vi "Build Slide Info.vi"(8 "error in (no error)":errorcluster, 11 "Parse Presentation in":refnum<class "Parse Presentation.lvclass">) -> (0 "error out":errorcluster, 3 "Parse Presentation out":refnum<class "Parse Presentation.lvclass">)   [LabVIEW 2015, in "Parse Presentation.lvclass"]
uses:
  Parse Presentation.lvclass
  Slide Info..cluster.ctl
  Parse Presentation.lvclass/Parse Presentation.ctl
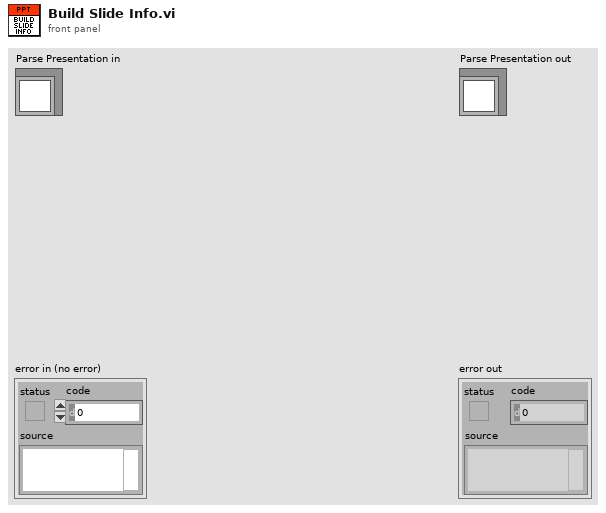
[diagram p1: front panel]
types:
  T1 = typedef "Parse Presentation.lvclass/Slide Info..cluster.ctl" = cluster{"Slide":i32, "Text":string, "Images":string}
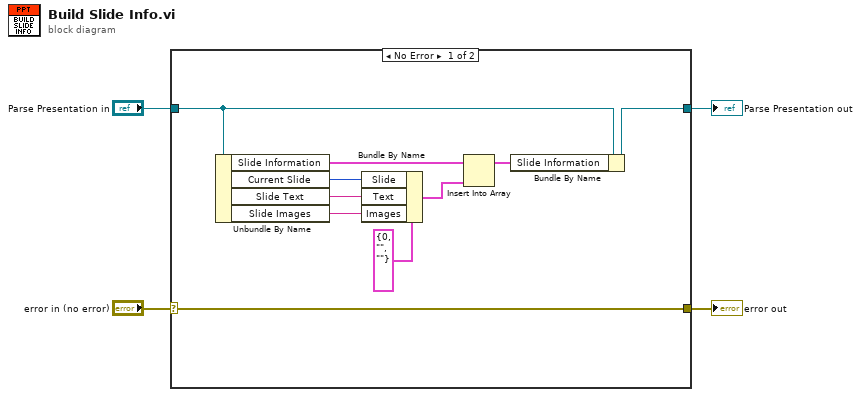
[diagram p0: block diagram]
diagram:
  n1 = case shown="No Error" "error in (no error)" {
    selector: "error in (no error)" -> [w14 w16]
    tunnel: [w14 w16] -> w3
    tunnel: [w12 w15] -> w1
    tunnel: "Parse Presentation in" -> [w13 w15]
    frame No Error {
      n2 = Unbundle By Name(w13) -> ("Slide Information"=w11:T1[], "Current Slide"=w9:i32, "Slide Text"=w8:string, "Slide Images"=w7:string)
      n3 = Bundle By Name(cluster=T1 {"Slide"=0, "Text"="", "Images"=""} ("Slide Information"), "Slide"=w9, "Text"=w8, "Images"=w7) -> (w5:T1)
      n4 = Insert Into Array(array=w11, new element=w5) -> (w10:T1[])  [unwired: 1 in]
      n5 = Bundle By Name(cluster=w13, "Slide Information"=w10) -> (w12:refnum<class "Parse Presentation.lvclass">)
    }
    frame Error {
    }
  }
  "error out" <- w3
  "Parse Presentation out" <- w1
